vi "Bulk Delete Wrapper.vi"(11 "Node Ptr":T1 format="%.0x") -> ()   [LabVIEW 2021, in "Modbus Master System Explorer.lvlib"]
uses:
  Modbus Master System Explorer.lvlib
  <vilib>/NI VeriStand/Custom Device API/Custom Device Item Ref.ctl
  <vilib>/NI VeriStand/Custom Device API/Custom Device API.lvlib
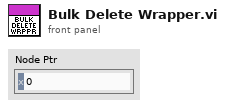
[diagram p1: front panel]
types:
  T1 = typedef "Custom Device API.lvlib/Custom Device Item Ref.ctl" = u64
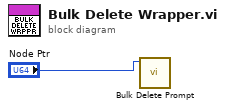
[diagram p0: block diagram]
diagram:
  n1 = call "Bulk Delete Prompt.vi"("Item Ref in"="Node Ptr") -> ()  [unwired: 10 in, 1 out]
